vi "Interpolation_Filter_Test.vi"() -> ()   [LabVIEW 2025]
uses:
  <vilib>/measure/maspectr.llb/Power Spectrum and PSD Export Mode.ctl
  <vilib>/measure/maspectr.llb/FFT Power Spectrum and PSD for 1 Chan.vi
  <vilib>/measure/NI_MAPro.lvlib
panel:
  out "original size":i32
  out "filtered size":i32
  out "Output valid":i16[](graph)
  out "filtered numeric":dbl[](array[numeric])
  out "Filtered signal":dbl[](graph)
  out "Power spectrum in":cluster{"f0":dbl, "df":dbl, "magnitude":dbl[]}(graph)
  out "Power spectrum out":cluster{"f0":dbl, "df":dbl, "magnitude":dbl[]}[](graph)
  out "Input signal":dbl[](graph)
  out "# of Iterations":i32
  out "# of samples":i32
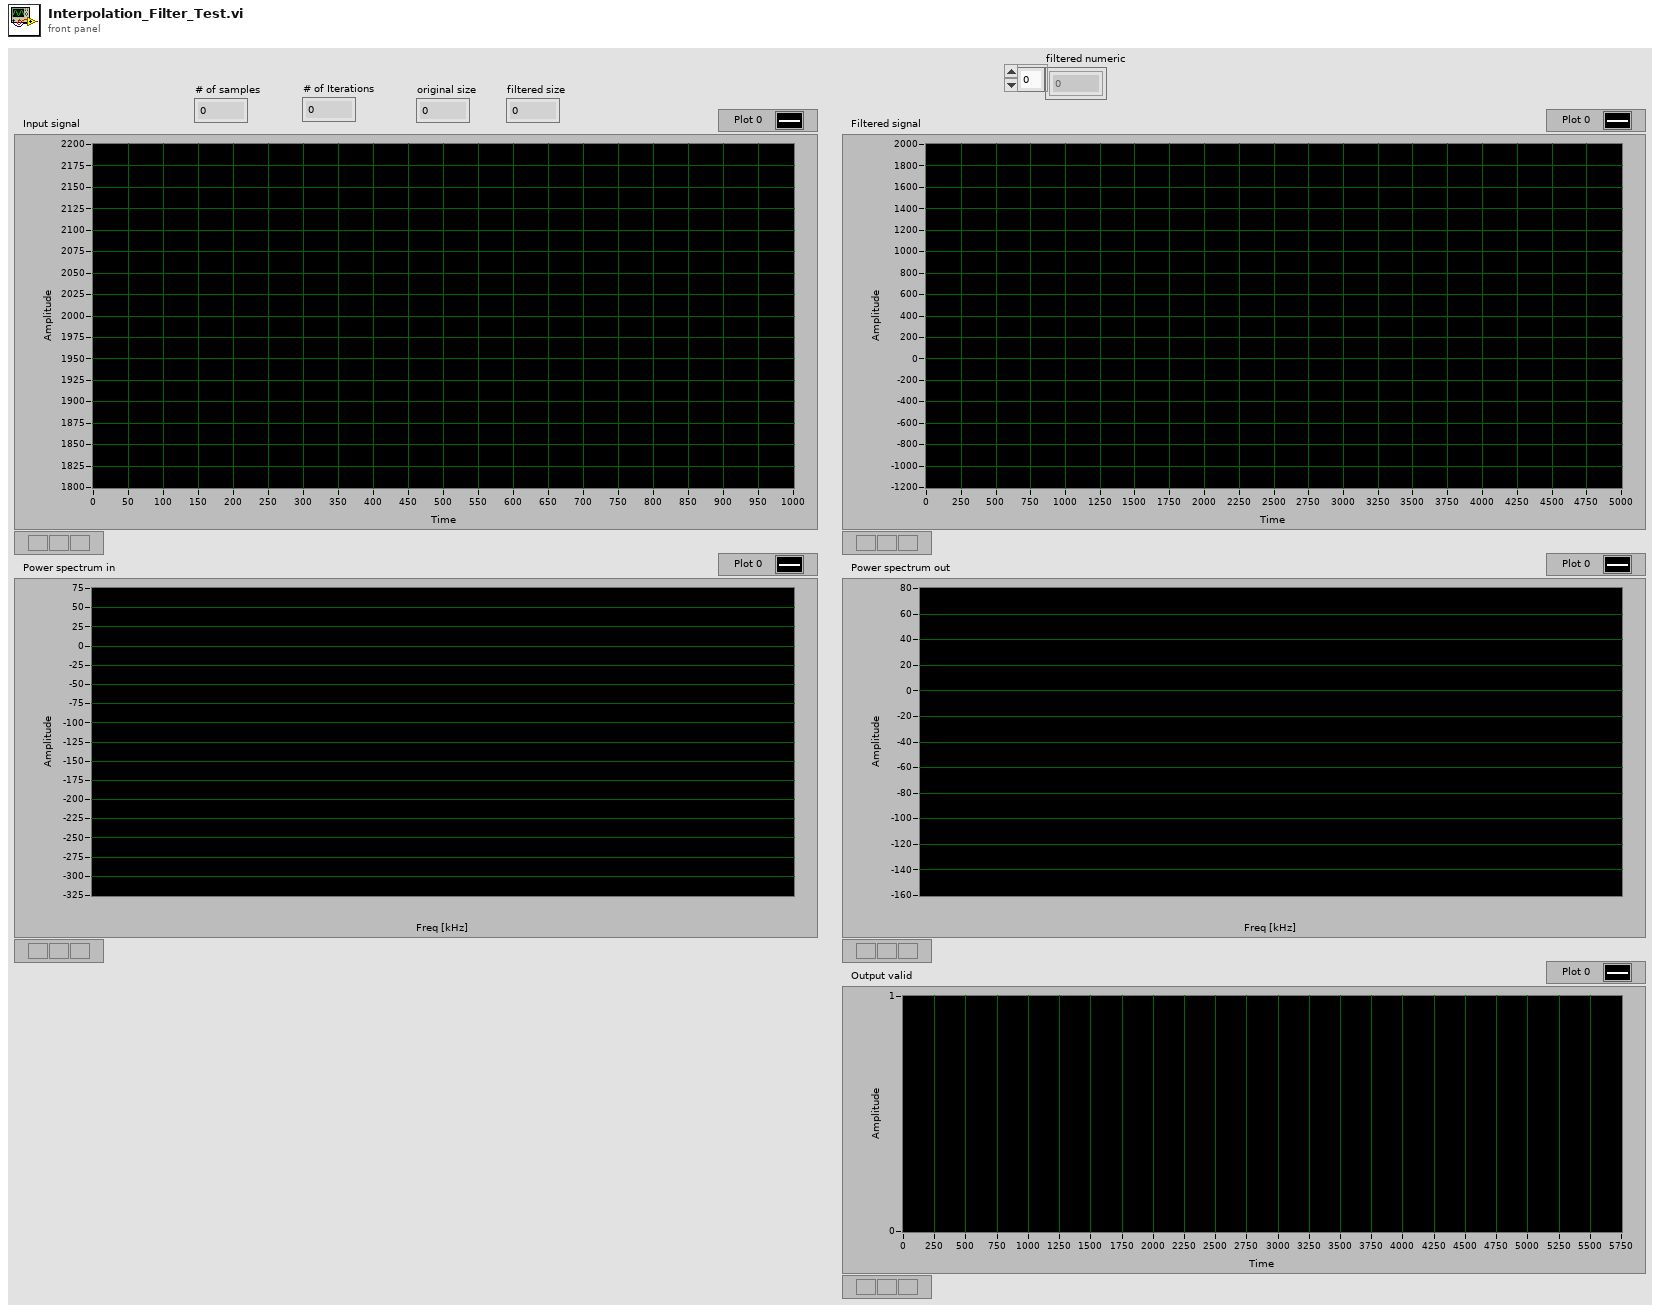
[diagram p1: front panel]
types:
  T1 = typedef "NI_MAPro.lvlib/Power Spectrum and PSD Export Mode.ctl" = u16
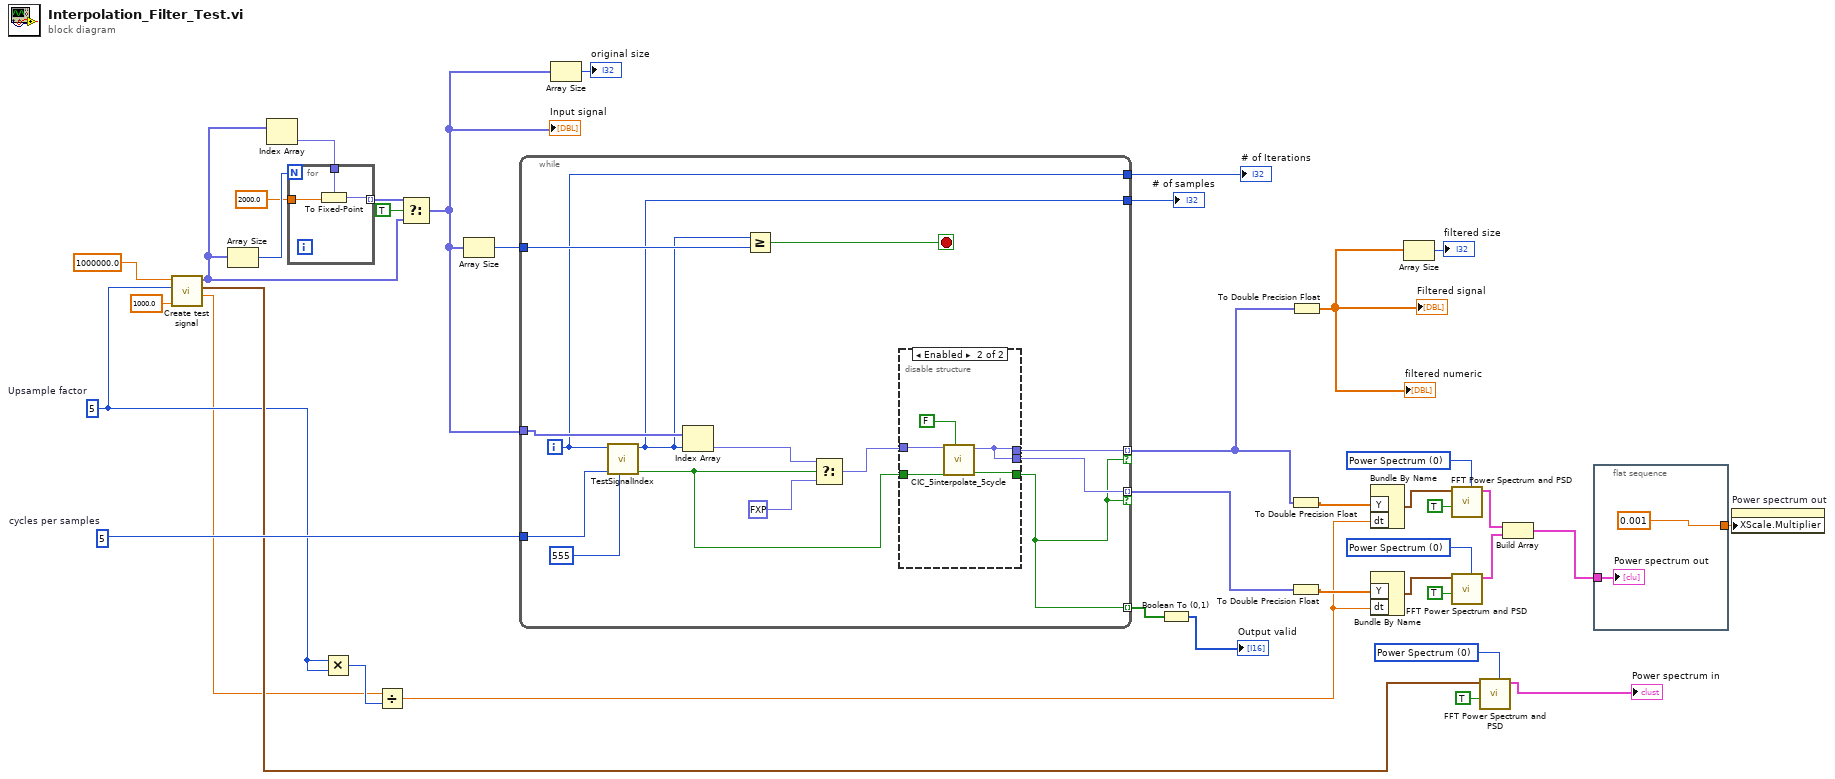
[diagram p0: block diagram]
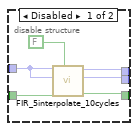
[diagram p2: hidden frame]
diagram:
  w24 = T1 0 items=["Power Spectrum", "Power Spectral Density"] ("export mode")
  w11 = 5  # Upsample factor
  w32 = 5  # cycles per samples
  w34 = T1 0 items=["Power Spectrum", "Power Spectral Density"] ("export mode")
  w38 = T1 0 items=["Power Spectrum", "Power Spectral Density"] ("export mode")
  n1 = call "Create test signal.vi"("Number of samples"=1000.0, "Downsample factor"=w11, "Sample rate"=1000000.0) -> ("dt"=w9:dbl, "signal out"=w30:waveform(dbl), "Y"=w3:fxp<+/-,16,14>[])  [unwired: 6 in]
  n2 = Array Size(array=w3) -> (size(s)=w6:i32)
  n3 = Index Array(array=w3) -> (element=w7:fxp<+/-,16,14>)  [unwired: 1 in]
  n4 = for {
    N: w6 -> [_]
    tunnel: w7 -> [w43]
    tunnel: 2000.0 ("Number of samples") -> [w42]
    tunnel: [w41] -> w4 mode=indexing
    n5 = To Fixed-Point(fixed-point type=w43, number=w42) -> (fixed-point=w41:fxp<+/-,16,14>)
  }
  n6 = Multiply(x=w11, y=w11) -> (x*y=w10:i32)
  n7 = Divide(x=w9, y=w10) -> (x/y=w8:dbl)
  n8 = Select(t=w4, s=TRUE, f=w3) -> (s? t:f=w2:fxp<+/-,16,14>[])
  "Input signal" <- w2
  n9 = Array Size(array=w2) -> (size(s)=w40:i32)
  n10 = while {
    tunnel: w2 -> [w57]
    tunnel: [w54] -> w21 mode=indexing if=w46
    tunnel: w40 -> [w55]
    tunnel: w32 -> [w53]
    tunnel: [w46] -> w31 mode=indexing
    tunnel: [w47] -> w20 mode=indexing if=w46
    tunnel: [w45] -> w14
    tunnel: [w44] -> w13
    i -> [w44]
    stop <- w56 stop-if-true
    n11 = call "TestSignalIndex.vi"("initial delay"=555, "cycles per sample"=w53, "index"=w44) -> ("valid out"=w48:bool, "array index"=w45:i32)  [unwired: 7 in]
    n12 = Index Array(array=w57, index=w45) -> (element=w52:fxp<+/-,16,14>)
    n13 = Greater Or Equal?(x=w45, y=w55) -> (x >= y?=w56:bool)
    n14 = Select(t=w52, s=w48, f=fxp<+/-,16,14> 0.0) -> (s? t:f=w51:fxp<+/-,16,14>)
    n15 = disable-structure shown="Enabled" {
      disable-tunnel: [w60 w64] -> w54
      disable-tunnel: w51 -> [w59 w68]
      disable-tunnel: w48 -> [w62 w66]
      disable-tunnel: [w58 w64] -> w47
      disable-tunnel: [w61 w65] -> w46
      frame Disabled {
        n16 = call "FIR_5interpolate_10cycles.vi"("reset"=FALSE, "valid in"=w62, "Q in"=w59, "I in"=w59) -> ("valid out"=w61:bool, "Q out"=w58:fxp<+/-,16,14>, "I out"=w60:fxp<+/-,16,14>)  [unwired: 4 in, 1 out]
      }
      frame Enabled {
        n17 = call "CIC_5interpolate_5cycle.vi"("reset"=FALSE, "valid in"=w66, "Data in"=w68) -> ("valid out"=w65:bool, "Data out"=w64:fxp<+/-,16,14>)  [unwired: 7 in]
      }
    }
  }
  "# of samples" <- w14
  "# of Iterations" <- w13
  n18 = Array Size(array=w2) -> (size(s)=→"original size":i32)
  n19 = Boolean To (0,1)(Boolean=w31) -> (0, 1=→"Output valid":i16[])
  n20 = To Double Precision Float(number=w21) -> (double precision float=w27:dbl[])
  n21 = To Double Precision Float(number=w20) -> (double precision float=w36:dbl[])
  n22 = To Double Precision Float(number=w21) -> (double precision float=w17:dbl[])
  "Filtered signal" <- w17
  "filtered numeric" <- w17
  n23 = Bundle By Name("Y"=w27, "dt"=w8) -> (w25:waveform(dbl))  [unwired: 1 in]
  n24 = Bundle By Name("Y"=w36, "dt"=w8) -> (w39:waveform(dbl))  [unwired: 1 in]
  n25 = Array Size(array=w17) -> (size(s)=→"filtered size":i32)
  n26 = call-poly <vilib>:"FFT Power Spectrum and PSD.vi"("export mode"=w24, "dB On (F)"=TRUE, "time signal"=w25) -> ("Power Spectrum / PSD"=w22:cluster{"f0":dbl, "df":dbl, "magnitude":dbl[]})  [unwired: 5 in, 3 out]
  n27 = call-poly <vilib>:"FFT Power Spectrum and PSD.vi"("export mode"=w38, "dB On (F)"=TRUE, "time signal"=w39) -> ("Power Spectrum / PSD"=w23:cluster{"f0":dbl, "df":dbl, "magnitude":dbl[]})  [unwired: 5 in, 3 out]
  n28 = call-poly <vilib>:"FFT Power Spectrum and PSD.vi"("export mode"=w34, "dB On (F)"=TRUE, "time signal"=w30) -> ("Power Spectrum / PSD"=→"Power spectrum in":cluster{"f0":dbl, "df":dbl, "magnitude":dbl[]})  [unwired: 5 in, 3 out]
  n29 = Build Array(w22, w23) -> (w19:cluster{"f0":dbl, "df":dbl, "magnitude":dbl[]}[])
  n30 = flat-sequence {
    tunnel: w19 -> [w70]
    tunnel: [0.001 ("X Scale.Offset and Multiplier:Multiplier")] -> w18
    frame #0 {
      "Power spectrum out" <- w70
    }
  }
  n31 = property on="Power spectrum out" class="WFGraph (strict)"("XScale.Multiplier"=w18) -> ()  [unwired: 2 in, 2 out]
